vi "abouttest.vi"() -> ()   [LabVIEW 2015]
panel:
  out "boards":u32
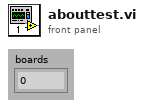
[diagram p1: front panel]
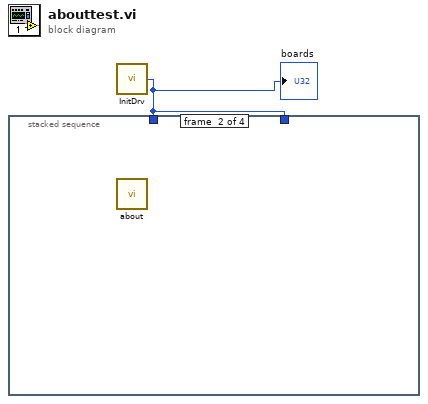
[diagram p0: block diagram]
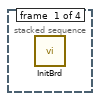
[diagram p2: hidden frame]
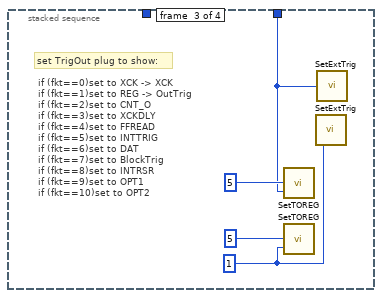
[diagram p3: hidden frame]
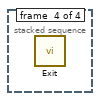
[diagram p4: hidden frame]
diagram:
  n1 = call "InitDrv.vi"() -> ("Boards"=w1:u8)  [unwired: 1 in]
  "boards" <- w1
  n2 = stacked-sequence {
    tunnel: w1 -> [_ _ _ _]
    tunnel: w1 -> [_ _ w3 _]
    frame #0 {
      n3 = call "InitBrd.vi"() -> ()  [unwired: 6 in]
    }
    frame #1 {
      n4 = call "about.vi"() -> ()  [unwired: 2 in]
    }
    frame #2 {
      w2 = u8 1
      # "set TrigOut plug to show:"
      # "if (fkt==0)set to XCK -> XCK\nif (fkt==1)set to REG -> OutTrig\nif (fkt==2)set to CNT_O\nif (fkt==3)set to XCKDLY\nif (fkt==4)set to FFREAD\nif (fkt==5)set to INTTRIG\nif (fkt==6)set to DAT\nif (fkt==7)set to BlockTrig\nif (fkt==8)set to INTRSR\nif (fkt==9)set to OPT1\nif (fkt==10)set to OPT2"
      n5 = call "SetTOREG.vi"("board"=w3, "fkt"=u8 5) -> ()  [unwired: 1 in]
      n6 = call "SetTOREG.vi"("board"=w2, "fkt"=u8 5) -> ()  [unwired: 1 in]
      n7 = call "SetExtTrig.vi"("boards"=w2) -> ()  [unwired: 1 in]
      n8 = call "SetExtTrig.vi"("boards"=w3) -> ()  [unwired: 1 in]
    }
    frame #3 {
      n9 = call "Exit.vi"() -> ()  [unwired: 1 in]
    }
  }
